vi "EnableSqWaveTest.vi"() -> ()   [LabVIEW 2011]
uses:
  subVIs/IFA300Command.ctl
panel:
  in  "Channel":i8=1
  in  "Port Name":string
  in  "Frequency":u8(slide) scale=0.0..5.0
  in  "Voltage":u8(slide) scale=0.0..3.0
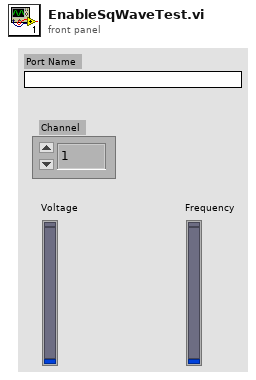
[diagram p1: front panel]
types:
  T1 = typedef "IFA300Command.ctl" = string
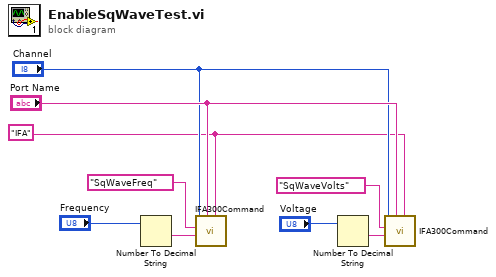
[diagram p0: block diagram]
diagram:
  w1 = "IFA" ("Channel Name")
  n1 = Number To Decimal String(number="Frequency") -> (decimal integer string=w6:string)  [unwired: 1 in]
  n2 = call "IFA300Command.vi"("Channel Name"=w1, "Port Name"="Port Name", "ValueToSet"=w6, "IFACommand"=T1 "SqWaveFreq", "Address"="Channel") -> ()  [unwired: 3 in, 3 out]
  n3 = Number To Decimal String(number="Voltage") -> (decimal integer string=w8:string)  [unwired: 1 in]
  n4 = call "IFA300Command.vi"("Channel Name"=w1, "Port Name"="Port Name", "ValueToSet"=w8, "IFACommand"=T1 "SqWaveVolts", "Address"="Channel") -> ()  [unwired: 3 in, 3 out]
